vi "DriveForDistance.vi"() -> ()   [LabVIEW 2017]
panel:
  in  "Distance":dbl
  in  "Speed":dbl
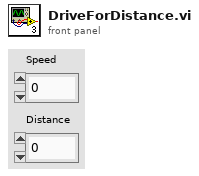
[diagram p1: front panel]
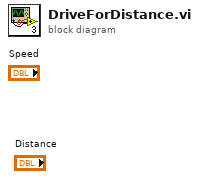
[diagram p0: block diagram]
diagram:
